vi "Save data file (stop) v2.vi"(11 "panel id":string) -> (0 "network file save error":errorcluster, 3 "file save path":string)   [LabVIEW 2013]
uses:
  program files/Global 1.vi
panel:
  out "C drive root path":string
  out "network file dir path":path
  out "network dir":string
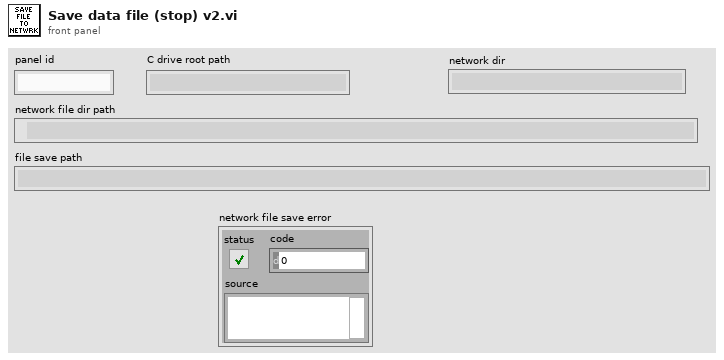
[diagram p1: front panel]
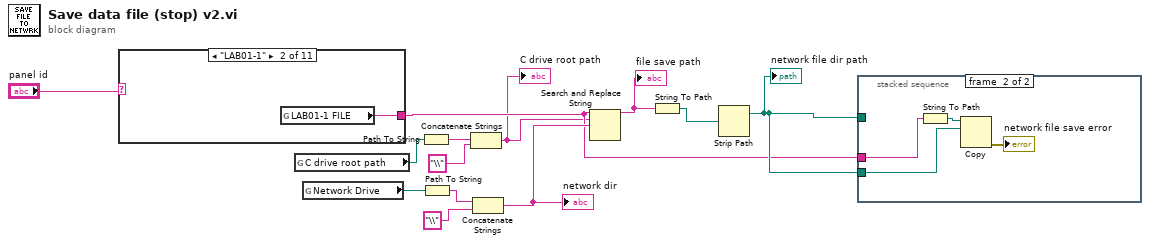
[diagram p0: block diagram]
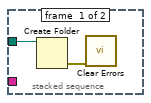
[diagram p2: hidden frame]
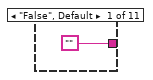
[diagram p3: hidden frame]
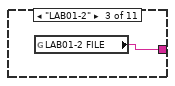
[diagram p4: hidden frame]
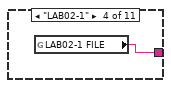
[diagram p5: hidden frame]
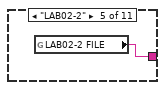
[diagram p6: hidden frame]
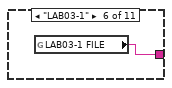
[diagram p7: hidden frame]
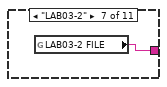
[diagram p8: hidden frame]
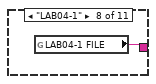
[diagram p9: hidden frame]
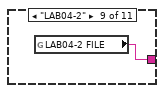
[diagram p10: hidden frame]
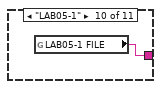
[diagram p11: hidden frame]
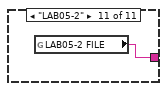
[diagram p12: hidden frame]
diagram:
  n1 = case shown="\"LAB01-1\"" "panel id" {
    tunnel: ["" w15 w16 w17 w18 w19 w20 w21 w22 w23 w24] -> w5
    frame "False", Default {
    }
    frame "LAB01-1" {
      n2 = global read "Global 1.vi" "LAB01-1 FILE"() -> (w15:string)
    }
    frame "LAB01-2" {
      n3 = global read "Global 1.vi" "LAB01-2 FILE"() -> (w16:string)
    }
    frame "LAB02-1" {
      n4 = global read "Global 1.vi" "LAB02-1 FILE"() -> (w17:string)
    }
    frame "LAB02-2" {
      n5 = global read "Global 1.vi" "LAB02-2 FILE"() -> (w18:string)
    }
    frame "LAB03-1" {
      n6 = global read "Global 1.vi" "LAB03-1 FILE"() -> (w19:string)
    }
    frame "LAB03-2" {
      n7 = global read "Global 1.vi" "LAB03-2 FILE"() -> (w20:string)
    }
    frame "LAB04-1" {
      n8 = global read "Global 1.vi" "LAB04-1 FILE"() -> (w21:string)
    }
    frame "LAB04-2" {
      n9 = global read "Global 1.vi" "LAB04-2 FILE"() -> (w22:string)
    }
    frame "LAB05-1" {
      n10 = global read "Global 1.vi" "LAB05-1 FILE"() -> (w23:string)
    }
    frame "LAB05-2" {
      n11 = global read "Global 1.vi" "LAB05-2 FILE"() -> (w24:string)
    }
  }
  n12 = global read "Global 1.vi" "C drive root path"() -> (w2:path)
  n13 = global read "Global 1.vi" "Network Drive"() -> (w12:path)
  n14 = Path To String(path=w2) -> (string=w3:string)
  n15 = Path To String(path=w12) -> (string=w11:string)
  n16 = Concatenate Strings(w3, "\\") -> (w1:string)
  "C drive root path" <- w1
  n17 = Concatenate Strings(w11, "\\") -> (w9:string)
  "network dir" <- w9
  n18 = Search and Replace String(input string=w5, search string=w1, replace string=w9) -> (result string=w8:string)  [unwired: 5 in, 3 out]
  "file save path" <- w8
  n19 = String To Path(string=w8) -> (path=w7:path)
  n20 = Strip Path(path=w7) -> (stripped path=w6:path)  [unwired: 1 out]
  "network file dir path" <- w6
  n21 = stacked-sequence {
    tunnel: w6 -> [w26 _]
    tunnel: w5 -> [_ w28]
    tunnel: w6 -> [_ w27]
    frame #0 {
      n22 = Create Folder(path (use dialog)=w26) -> (error out=w25:errorcluster)  [unwired: 2 in, 2 out]
      n23 = call <vilib>:"Clear Errors.vi"("error in (no error)"=w25) -> ()  [unwired: 6 in, 1 out]
    }
    frame #1 {
      n24 = String To Path(string=w28) -> (path=w29:path)
      n25 = Copy(10:w27, 11:w29) -> (0:→"network file save error":errorcluster)  [unwired: 3 in, 2 out]
    }
  }
